vi "Withdraw.vi"(8 "error in (no error)":errorcluster, 10 "Amount":dbl, 11 "SimpleExpenseAccount in":refnum<class "SimpleExpenseAccount.lvclass">) -> (0 "error out":errorcluster, 1 "Success?":bool, 2 "Balance":dbl, 3 "SimpleExpenseAccount out":refnum<class "SimpleExpenseAccount.lvclass">)   [LabVIEW 2020, in "SimpleExpenseAccount.lvclass"]
uses:
  SimpleExpenseAccount.lvclass
  SimpleExpenseAccount.lvclass/SimpleExpenseAccount.ctl
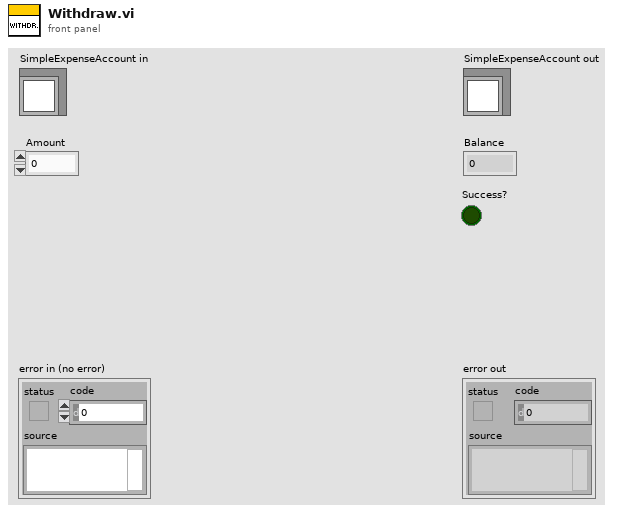
[diagram p1: front panel]
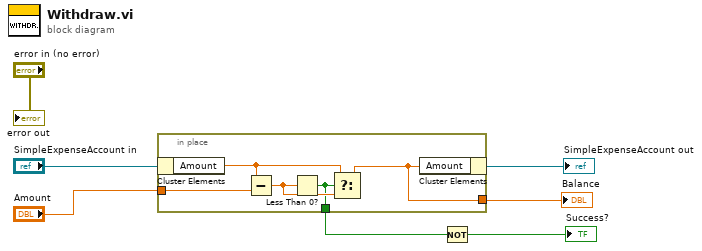
[diagram p0: block diagram]
diagram:
  n1 = in-place {
    in-place-border: "Amount" -> [w12]
    in-place-border: [w9] -> w3
    in-place-border: [w8] -> w2
    n2 = in-place-cluster #1("SimpleExpenseAccount in") -> ("Amount"=w10:dbl)
    n3 = Subtract(x=w10, y=w12) -> (x-y=w11:dbl)
    n4 = Less Than 0?(x=w11) -> (x < 0?=w8:bool)
    n5 = Select(t=w10, s=w8, f=w11) -> (s? t:f=w9:dbl)
    n6 = in-place-cluster #1("Amount"=w9) -> (→"SimpleExpenseAccount out":refnum<class "SimpleExpenseAccount.lvclass">)
  }
  "Balance" <- w3
  n7 = Not(x=w2) -> (.not. x?=→"Success?":bool)
  "error out" <- "error in (no error)"
